vi "Set Magnet Field.vi"(4 "Axis":T1, 6 "Mode":T2, 8 "error in (no error)":errorcluster, 9 "Target Rate (T/min)":dbl, 10 "Target Field (T)":dbl, 11 "Instrument.Oxford1820 in":refnum<class "Instrument.Oxford1820.lvclass">) -> (0 "error out":errorcluster, 3 "Instrument.Oxford1820 out":refnum<class "Instrument.Oxford1820.lvclass">)   [LabVIEW 2016, in "Instrument.Oxford1820.lvclass"]
uses:
  Instrument.Oxford1820.lvclass
  <userlib>/LevyLab/Levylab Instruments/Instrument Types/Cryostat/Typedefs/Magnet Mode--Enum.ctl
  <userlib>/LevyLab/Levylab Instruments/Instrument Types/Cryostat/Typedefs/Magnet Axis--Enum.ctl
  <userlib>/LevyLab/Oxford 1820 API/Typedefs/Targets.ctl
  <userlib>/LevyLab/Oxford 1820 API/Mercury-1820-API.lvlib
  <userlib>/LevyLab/Levylab Instruments/Instrument Types/Cryostat/Instrument.Cryostat.lvclass
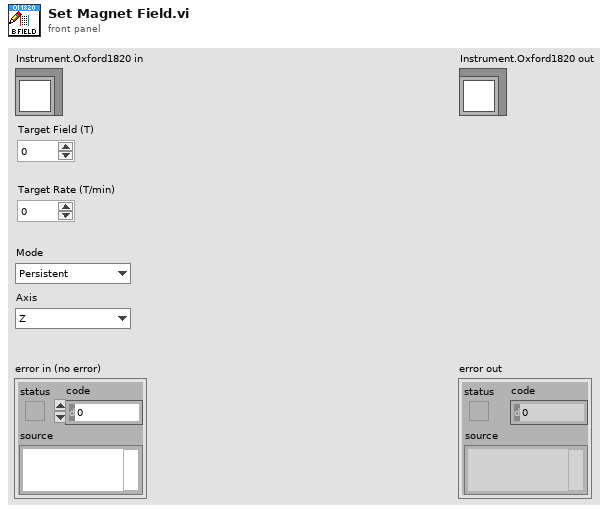
[diagram p1: front panel]
types:
  T1 = typedef "Instrument.Cryostat.lvclass/Magnet Axis--Enum.ctl" = enum16{"Z", "X", "Y"}
  T2 = typedef "Instrument.Cryostat.lvclass/Magnet Mode--Enum.ctl" = enum16{"Persistent", "Driven"}
  T3 = typedef "Mercury-1820-API.lvlib/Targets.ctl" = cluster{"Target Field (T)":dbl, "Target Field Rate (T/min)":dbl}
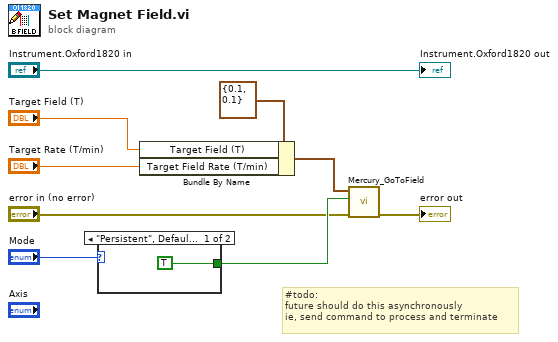
[diagram p0: block diagram]
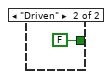
[diagram p2: hidden frame]
diagram:
  # "#todo:\nfuture should do this asynchronously\nie, send command to process and terminate"
  n1 = case shown="\"Persistent\", Default" "Mode" {
    tunnel: [TRUE ("persistent mode") FALSE ("persistent mode")] -> w5
    frame "Persistent", Default {
    }
    frame "Driven" {
    }
  }
  n2 = Bundle By Name(cluster=T3 {"Target Field (T)"=0.1, "Target Field Rate (T/min)"=0.1} ("Mercury Targets"), "Target Field (T)"="Target Field (T)", "Target Field Rate (T/min)"="Target Rate (T/min)") -> (w3:T3)
  n3 = call <userlib>:"Mercury_GoToField.vi"("error in"="error in (no error)", "persistent mode"=w5, "Mercury Targets"=w3) -> ("error out"=→"error out":errorcluster)  [unwired: 8 in]
  "Instrument.Oxford1820 out" <- "Instrument.Oxford1820 in"
